vi "close all.vi"(8 "error in (no error)":errorcluster, 11 "pulse_gen_and_detect_p2p in":refnum<class "pulse_gen_and_detect_p2p.lvclass">) -> (0 "error out":errorcluster, 3 "pulse_gen_and_detect_p2p out":refnum<class "pulse_gen_and_detect_p2p.lvclass">)   [LabVIEW 2021, in "pulse_gen_and_detect_p2p.lvclass"]
uses:
  pulse_gen_and_detect_p2p.lvclass
  pulse_gen_and_detect_p2p.lvclass/pulse_gen_and_detect_p2p.ctl
  <vilib>/FPGAPlugInAG/Dynamic/niLvFpga_Close_Dynamic.vi
  <vilib>/rvi/interface/nirviCloseFPGA/nirviCloseFPGA.xnode
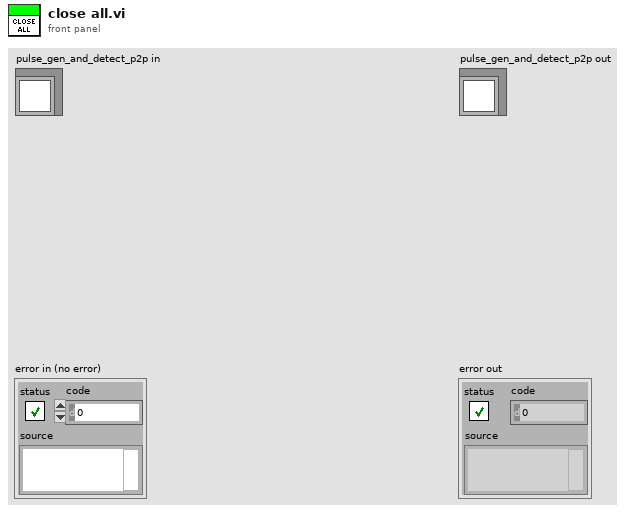
[diagram p1: front panel]
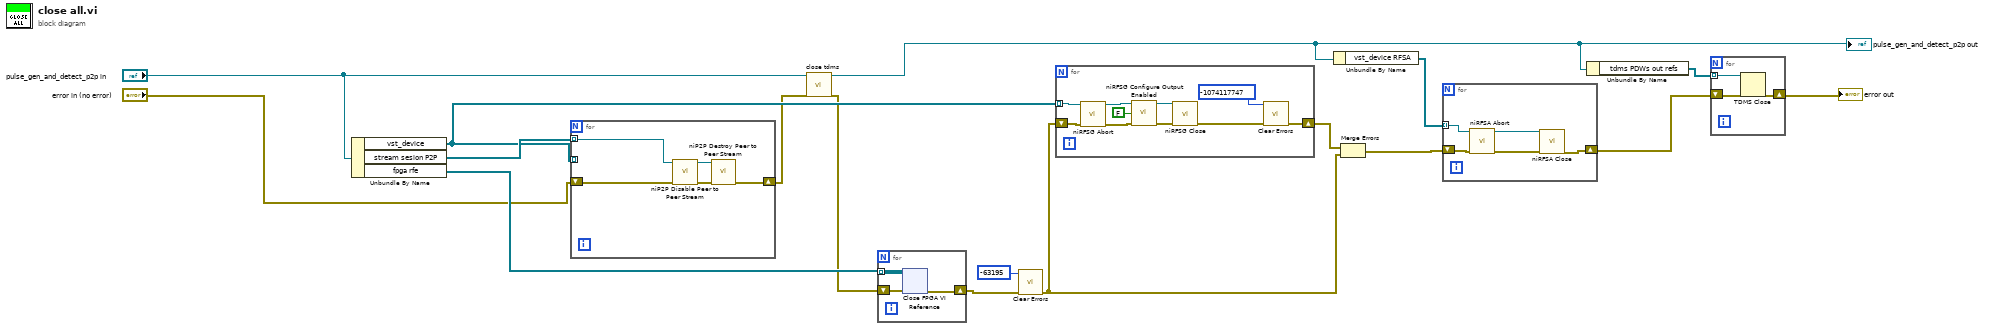
[diagram p0: block diagram]
diagram:
  n1 = Unbundle By Name("pulse_gen_and_detect_p2p in") -> ("vst_device"=w13:refnum<k15>[], "stream sesion P2P"=w14:refnum<k20>[], "fpga rfe"=w17:refnum<k20>[])
  n2 = for {
    tunnel: w14 -> [w19] mode=indexing
    shift-right: [w20] -> w10
    shift-left: "error in (no error)" -> [w18]
    tunnel: w13 -> [_] mode=indexing
    n3 = call <vilib>:"niP2P Disable Peer to Peer Stream.vi"("stream session"=w19, "error in (no error)"=w18) -> ("stream session out"=w22:refnum<k20>, "error out"=w21:errorcluster)  [unwired: 12 in]
    n4 = call <vilib>:"niP2P Destroy Peer to Peer Stream.vi"("stream session"=w22, "error in (no error)"=w21) -> ("error out"=w20:errorcluster)  [unwired: 13 in]
  }
  n5 = call-dynamic "close tdms.vi"("error in (no error)"=w10, "device_type in"="pulse_gen_and_detect_p2p in") -> ("error out"=w9:errorcluster, "device_type out"=w3:refnum<class "pulse_gen_and_detect_p2p.lvclass">)  [unwired: 8 in]
  "pulse_gen_and_detect_p2p out" <- w3
  n6 = for {
    shift-right: [w24] -> w15
    shift-left: w9 -> [w25]
    tunnel: w17 -> [w23] mode=indexing
    n7 = xnode "Close FPGA VI Reference"("FPGA VI Reference In"=w23, "error in"=w25) -> ("error out"=w24:errorcluster)
  }
  n8 = call <vilib>:"Clear Errors.vi"("error in (no error)"=w15, "specific error code to clear (0: all)"=-63195) -> ("error out"=w12:errorcluster)  [unwired: 4 in, 1 out]
  n9 = for {
    tunnel: w13 -> [w29] mode=indexing
    shift-right: [w30] -> w11
    shift-left: w12 -> [w28]
    n10 = call <instrlib>:"niRFSG Abort.vi"("instrument handle"=w29, "error in"=w28) -> ("instrument handle out"=w26:refnum<k15>, "error out"=w27:errorcluster)  [unwired: 12 in]
    n11 = call <instrlib>:"niRFSG Configure Output Enabled.vi"("instrument handle"=w26, "output enabled"=FALSE, "error in"=w27) -> ("instrument handle out"=w34:refnum<k15>, "error out"=w35:errorcluster)  [unwired: 11 in]
    n12 = call <instrlib>:"niRFSG Close.vi"("instrument handle"=w34, "error in"=w35) -> ("error out"=w31:errorcluster)  [unwired: 13 in]
    n13 = call <vilib>:"Clear Errors.vi"("error in (no error)"=w31, "specific error code to clear (0: all)"=-1074117747) -> ("error out"=w30:errorcluster)  [unwired: 4 in, 1 out]
  }
  n14 = Unbundle By Name(w3) -> ("vst_device RFSA"=w5:refnum<k15>[])
  n15 = Merge Errors(w11, w12) -> (w6:errorcluster)
  n16 = for {
    tunnel: w5 -> [w36] mode=indexing
    shift-right: [w37] -> w2
    shift-left: w6 -> [w39]
    n17 = call <instrlib>:"niRFSA Abort.vi"("instrument handle"=w36, "error in"=w39) -> ("instrument handle out"=w40:refnum<k15>, "error out"=w38:errorcluster)  [unwired: 12 in]
    n18 = call <instrlib>:"niRFSA Close.vi"("instrument handle"=w40, "error in"=w38) -> ("error out"=w37:errorcluster)  [unwired: 13 in]
  }
  n19 = Unbundle By Name(w3) -> ("tdms PDWs out refs"=w4:refnum<k34>[])
  n20 = for {
    shift-right: [w42] -> w1
    shift-left: w2 -> [w43]
    tunnel: w4 -> [w41] mode=indexing
    n21 = TDMS Close(8:w43, 11:w41) -> (0:w42:errorcluster)  [unwired: 1 out]
  }
  "error out" <- w1
